vi "DailyEnd.vi"   [LabVIEW 2015]
uses:
  <userlib>/Newport ESP301/Newport ESP301.lvlib
panel:
  # "Run this at the end of the day to make \nsure you dont have to rerun the setup program"
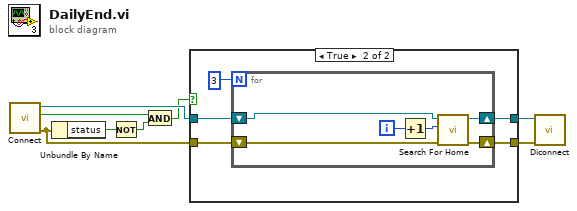
[diagram p0: block diagram]
diagram:
  n1 = call "Connect.vi"() -> ("error out"=w3:errorcluster, "Connected"=w6:bool, "VISA resource name out"=w8:refnum<visa-resource-name>)  [unwired: 5 in]
  n2 = Unbundle By Name(w3) -> ("status"=w7:bool)
  n3 = Not(x=w7) -> (.not. x?=w5:bool)
  n4 = And(x=w6, y=w5) -> (x .and. y?=w4:bool)
  n5 = case shown="True" w4 {
    tunnel: w8 -> [w10 w12]
    tunnel: w3 -> [w9 w13]
    tunnel: [w10 w15] -> w2
    tunnel: [w9 w14] -> w1
    frame False {
    }
    frame True {
      n6 = for {
        N: 3 -> [_]
        shift-right: [w18] -> w15
        shift-left: w12 -> [w19]
        shift-right: [w17] -> w14
        shift-left: w13 -> [w20]
        i -> [w21]
        n7 = Increment(x=w21) -> (x+1=w16:i32)
        n8 = call <userlib>:"Search For Home.vi"("error in (no error)"=w20, "Axis (1)"=w16, "VISA resource name"=w19) -> ("error out"=w17:errorcluster, "VISA resource name out"=w18:refnum<visa-resource-name>)  [unwired: 4 in]
      }
    }
  }
  n9 = call "Diconnect.vi"("error in (no error)"=w1, "VISA resource name"=w2) -> ()  [unwired: 6 in]
